vi "Configure CSV.vi"(6 "Original CSV Format":enum16{"Format A", "Format B"}(ring)=enum."Format B", 8 "error in (no error)":errorcluster, 9 "Run Mode Est Settings":refnum<notifier>, 10 "All Terminal Data":T1(array[cluster]), 11 "Settings IN":T2={"State"=enum."Idle", "Settings"="", "Online"=FALSE, "S3DK"={"Signals"={"Phasor"=[], "Analog"=[], "Digital"=[]}}, "CSV"={"Index"=0, "Parcel Length"=0, "EOF?"=FALSE, "Config"={"Mode"=enum."Full timestamp", "delimiter (\\t)"="\t", "Path"=path "", "Rectangular?"=FALSE}}}) -> (0 "error out":errorcluster, 1 "Remaining Terminal Data":T1(array[cluster]), 3 "Settings OUT":T2={"State"=enum."Idle", "Settings"="", "Online"=FALSE, "S3DK"={"Signals"={"Phasor"=[], "Analog"=[], "Digital"=[]}}, "CSV"={"Index"=0, "Parcel Length"=0, "EOF?"=FALSE, "Config"={"Mode"=enum."Full timestamp", "delimiter (\\t)"="\t", "Path"=path "", "Rectangular?"=FALSE}}})   [LabVIEW 2017, in "Acquisition.lvlib"]
doc: "Configure the hardware."
uses:
  Acquisition.lvlib
  Acquisition Settings.ctl
  Acquisition State.ctl
  support/libs/CSV Reader/Mode CSV reader.ctl
panel:
  in  "OK Button":bool
  in  "Terminal Selection":u16(ring) items=["0 - Terminal A", "1 - Terminal B", "2 - Terminal C", "6 - Terminal D"]
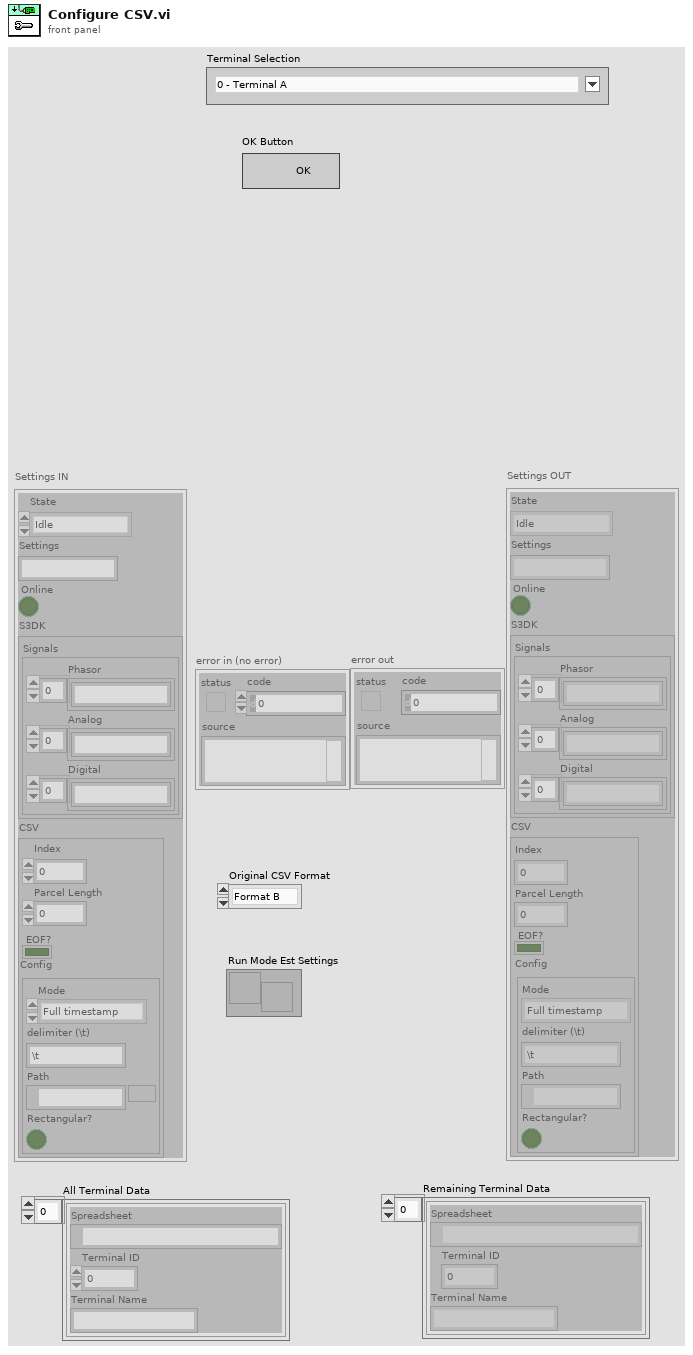
[diagram p1: front panel]
types:
  T1 = cluster{"Spreadsheet":path, "Terminal ID":u32, "Terminal Name":string}[]
  T2 = typedef "Acquisition.lvlib/Acquisition Settings.ctl" = cluster{"State":T3, "Settings":string, "Online":bool, "S3DK":cluster{"Signals":cluster{"Phasor":string[], "Analog":string[], "Digital":string[]}}, "CSV":cluster{"Index":i32, "Parcel Length":i32, "EOF?":bool, "Config":cluster{"Mode":T4, "delimiter (\\t)":string, "Path":path, "Rectangular?":bool}}}
  T3 = typedef "Acquisition.lvlib/Acquisition State.ctl" = enum16{"Idle", "Idle S3DK", "Acquiring S3DK", "Idle CSV", "Acquiring CSV"}
  T4 = typedef "Mode CSV reader.ctl" = enum16{"Full timestamp", "Relative Time", "Seconds Time", "Nanoseconds Time"}
  T5 = cluster{"Spreadsheet":path, "Terminal ID":u32, "Terminal Name":string}
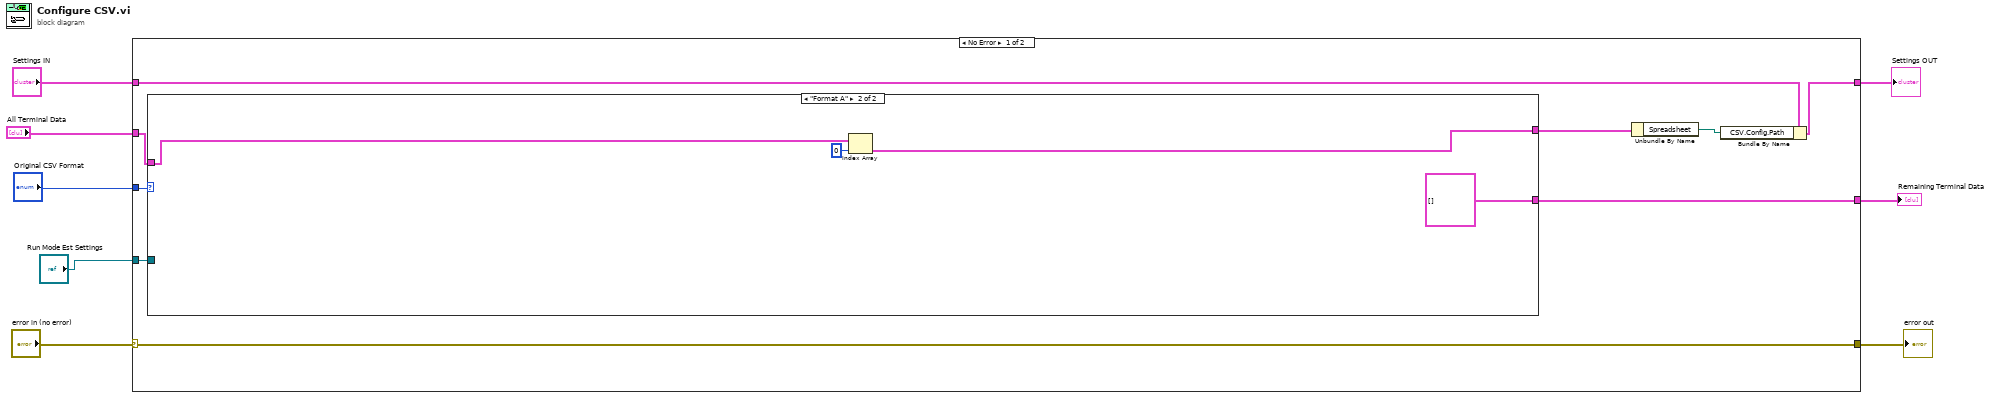
[diagram p0: block diagram]
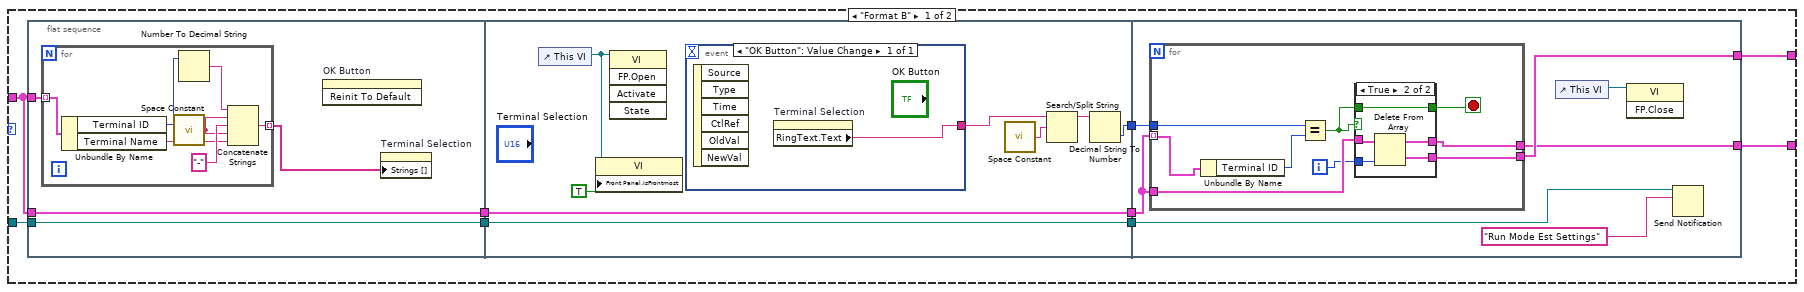
[diagram p2: hidden frame]
diagram:
  n1 = case shown="No Error" "error in (no error)" {
    selector: "error in (no error)" -> [w17 w74]
    tunnel: [w17 w74] -> w7
    tunnel: "Settings IN" -> [w16 w75]
    tunnel: [w15 w75] -> w5
    tunnel: "All Terminal Data" -> [w10 w73]
    tunnel: "Original CSV Format" -> [w12 _]
    tunnel: "Run Mode Est Settings" -> [w11 _]
    tunnel: [w9 w73] -> w1
    frame No Error {
      n2 = case shown="\"Format A\"" w12 {
        tunnel: [w23 w70] -> w14
        tunnel: w10 -> [w19 w72]
        tunnel: w11 -> [w20 _]
        tunnel: [w18 T1 [] ("All Terminal Data")] -> w9
        frame "Format B" {
          n3 = flat-sequence {
            tunnel: w19 -> [w30]
            tunnel: [w29] -> w26
            tunnel: w19 -> [w29]
            tunnel: [w27] -> w21
            tunnel: w20 -> [w27]
            tunnel: w26 -> [w45]
            tunnel: [w45] -> w25
            tunnel: [w41] -> w24
            tunnel: [w38] -> w22
            tunnel: w21 -> [w38]
            tunnel: w25 -> [w49]
            tunnel: [w53] -> w23
            tunnel: w24 -> [w52]
            tunnel: w22 -> [w50]
            tunnel: [w48] -> w18
            frame #0 {
              n4 = for {
                tunnel: w30 -> [w31] mode=indexing
                tunnel: [w32] -> w28 mode=indexing
                n5 = Unbundle By Name(w31) -> ("Terminal ID"=w37:u32, "Terminal Name"=w34:string)
                n6 = call <vilib>:"Space Constant.vi"() -> ("String"=w33:string)
                n7 = Number To Decimal String(number=w37) -> (decimal integer string=w36:string)  [unwired: 1 in]
                n8 = Concatenate Strings(w36, w33, "-", w33, w34) -> (w32:string)
              }
              n9 = invoke on="OK Button" class="Bool" method="Reinit To Default"() -> ()  [unwired: 3 in, 3 out]
              n10 = property on="Terminal Selection" class="Ring (strict)"("Strings []"=w28) -> ()  [unwired: 2 in, 2 out]
            }
            frame #1 {
              n11 = control-ref of="This VI"() -> (w40:refnum<vi>)
              n12 = property class="VI"(reference=w40, "Front Panel.IsFrontmost"=TRUE ("Front Panel Window:Is Frontmost")) -> ()  [unwired: 1 in, 2 out]
              n13 = invoke class="VI" method="FP.Open"(reference=w40) -> ()  [unwired: 4 in, 5 out]
              n14 = event shown="[0] \"OK Button\": Value Change" {
                selector: _ -> [_]
                dyn-events: _ -> [_]
                timeout: _ -> [_]
                tunnel: [w46] -> w43
                event "OK Button": Value Change {
                  n15 = event-data() -> ()  [unwired: 1 in, 6 out]
                  n16 = property on="Terminal Selection" class="Ring (strict)"() -> ("RingText.Text"=w46:string)  [unwired: 2 in, 2 out]
                }
              }
              n17 = call <vilib>:"Space Constant.vi"() -> ("String"=w44:string)
              n18 = Search/Split String(string=w43, search string/char (-)=w44) -> (substring before match=w42:string)  [unwired: 1 in, 2 out]
              n19 = Decimal String To Number(string=w42) -> (number=w41:i32)  [unwired: 2 in, 1 out]
            }
            frame #2 {
              n20 = for {
                tunnel: w49 -> [w61] mode=indexing
                tunnel: [w58] -> w53
                tunnel: w52 -> [w62]
                tunnel: w49 -> [w59]
                tunnel: [w57] -> w48
                i -> [w56]
                stop <- w54 stop-if-true
                n21 = Unbundle By Name(w61) -> ("Terminal ID"=w60:u32)
                n22 = Equal?(x=w62, y=w60) -> (x = y?=w55:bool)
                n23 = case shown="True" w55 {
                  tunnel: w59 -> [_ w68]
                  tunnel: [_ w67] -> w58
                  tunnel: [_ w66] -> w57
                  tunnel: w56 -> [_ w65]
                  tunnel: w55 -> [w63 w64]
                  tunnel: [w63 w64] -> w54
                  frame False {
                  }
                  frame True {
                    n24 = Delete From Array(array=w68, index=w65) -> (deleted portion=w67:T5, array with subset deleted=w66:T1)  [unwired: 1 in]
                  }
                }
              }
              n25 = control-ref of="This VI"() -> (w47:refnum<vi>)
              n26 = invoke class="VI" method="FP.Close"(reference=w47) -> ()  [unwired: 2 in, 3 out]
              n27 = Send Notification(notification="Run Mode Est Settings", notifier=w50) -> ()  [unwired: 1 in, 2 out]
            }
          }
        }
        frame "Format A" {
          n28 = Index Array(array=w72, index=0) -> (element=w70:T5)
        }
      }
      n29 = Unbundle By Name(w14) -> ("Spreadsheet"=w13:path)
      n30 = Bundle By Name(cluster=w16, "CSV.Config.Path"=w13) -> (w15:T2)
    }
    frame Error {
    }
  }
  "Settings OUT" <- w5
  "error out" <- w7
  "Remaining Terminal Data" <- w1
